vi "Compile Fully Custom Teeth.vi"(7 "Custom Device Ref":T1 format="%.0x", 8 "error in (no error)":errorcluster, 10 "Channel Descriptors in":T2, 11 "Fully custom teeth refs":T1[](array[typedef]) format="%.0x") -> (0 "error out":errorcluster, 2 "Channel Descriptors out":T2, 4 "Fully Custom Teeth":T9[](array[typedef]))   [LabVIEW 2011, in "Engine Sim System Explorer.lvlib"]
uses:
  Engine Sim System Explorer.lvlib
  <vilib>/NI Veristand/Custom Device API/Custom Device API.lvlib
  <vilib>/NI Veristand/Custom Device API/Get Item Property (U16).vi
  <vilib>/NI Veristand/Custom Device API/Get Item Property (Variant).vi
  <vilib>/NI Veristand/Custom Device API/Get Item Property (Boolean).vi
  Shared/Engine Simulation Global.vi
  Engine Simulation Shared.lvlib
  Shared/FullyCustomProfileConfig.ctl
  Shared/FullyCustomCommMode.ctl
  Shared/FullyCustomConfig.ctl
  <vilib>/NI Veristand/Custom Device API/Custom Device Item Ref.ctl
  Shared/InputChannelTypes.ctl
  <vilib>/rvi/DataTransferAndStorage/Container/Common/niFpgaDataTypeControl.ctl
  Shared/FPGA Write Descriptor.ctl
  Shared/OutputChannelTypes.ctl
  Shared/FPGA Read Descriptor.ctl
  Shared/Channel Descriptors.ctl
  Shared/Status Chan Descriptor.ctl
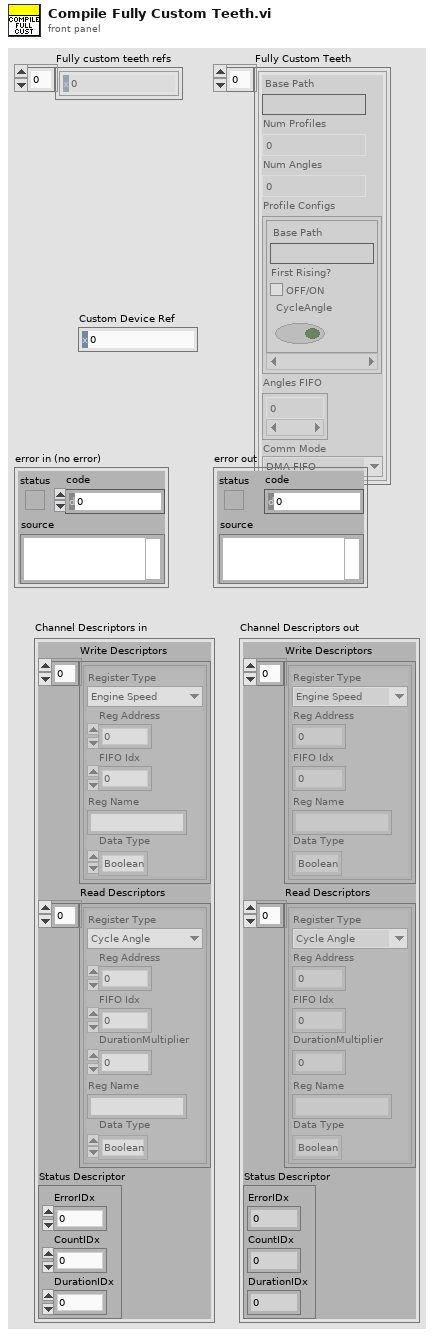
[diagram p1: front panel]
types:
  T1 = typedef "Custom Device API.lvlib/Custom Device Item Ref.ctl" = u64
  T2 = typedef "Engine Simulation Shared.lvlib/Channel Descriptors.ctl" = cluster{"Write Descriptors":T3[], "Read Descriptors":T6[], "Status Descriptor":T8}
  T3 = typedef "Engine Simulation Shared.lvlib/FPGA Write Descriptor.ctl" = cluster{"Register Type":T4, "Reg Address":u32, "FIFO Idx":i32, "Reg Name":string, "Data Type":T5}
  T4 = typedef "Engine Simulation Shared.lvlib/InputChannelTypes.ctl" = enum16{"Engine Speed", "Offset"}
  T5 = typedef "niFpgaDataTypeControl.ctl" = enum32{"Boolean", "I8", "I16", "I32", "I64", "U8", "U16", "U32", "U64", "FXP", "CustomControl"}
  T6 = typedef "Engine Simulation Shared.lvlib/FPGA Read Descriptor.ctl" = cluster{"Register Type":T7, "Reg Address":u32, "FIFO Idx":i32, "DurationMultiplier":dbl, "Reg Name":string, "Data Type":T5}
  T7 = typedef "Engine Simulation Shared.lvlib/OutputChannelTypes.ctl" = enum16{"Cycle Angle", "Crank Angle", "Time Duration", "Angle Duration", "Start Angle", "End Angle"}
  T8 = typedef "Engine Simulation Shared.lvlib/Status Chan Descriptor.ctl" = cluster{"ErrorIDx":i32, "CountIDx":i32, "DurationIDx":i32}
  T9 = typedef "Engine Simulation Shared.lvlib/FullyCustomConfig.ctl" = cluster{"Base Path":string, "Num Profiles":u8, "Num Angles":u8, "Profile Configs":T10[], "Angles FIFO":u64[], "Comm Mode":T11}
  T10 = typedef "Engine Simulation Shared.lvlib/FullyCustomProfileConfig.ctl" = cluster{"Base Path":string, "First Rising?":bool, "CycleAngle":bool}
  T11 = typedef "Engine Simulation Shared.lvlib/FullyCustomCommMode.ctl" = enum16{"DMA FIFO", "FP Data Transfer"}
  T12 = typedef "Custom Device API.lvlib/Custom Device Item Info.ctl" = cluster{"Name":string, "Is Channel":bool, "GUID":string}
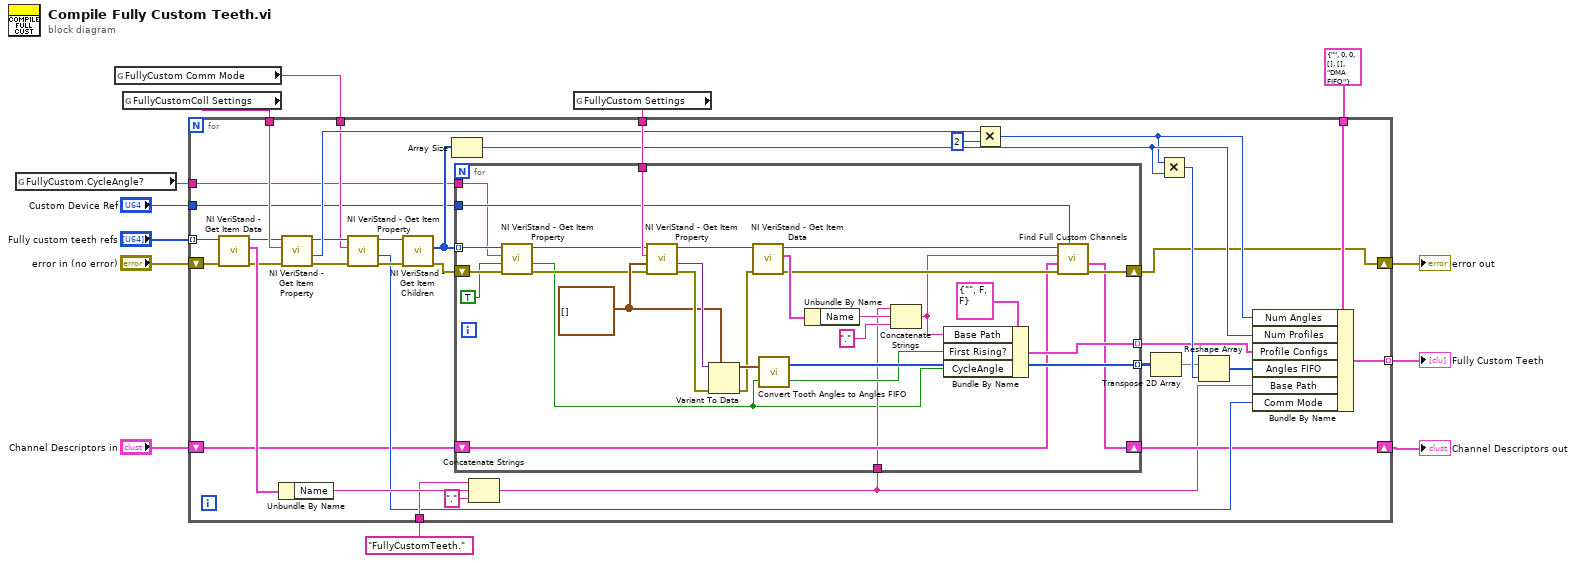
[diagram p0: block diagram]
diagram:
  n1 = global read "Engine Simulation Global.vi" "FullyCustom.CycleAngle?"() -> (w13:string)
  n2 = global read "Engine Simulation Global.vi" "FullyCustom Comm Mode"() -> (w12:string)
  n3 = global read "Engine Simulation Global.vi" "FullyCustomColl Settings"() -> (w6:string)
  n4 = global read "Engine Simulation Global.vi" "FullyCustom Settings"() -> (w7:string)
  n5 = for {
    shift-right: [w19] -> w10
    shift-left: "error in (no error)" -> [w41]
    tunnel: "Fully custom teeth refs" -> [w40] mode=indexing
    tunnel: w6 -> [w48]
    tunnel: w7 -> [w46]
    tunnel: T9 {"Base Path"="", "Num Profiles"=0, "Num Angles"=0, "Profile Configs"=[], "Angles FIFO"=[], "Comm Mode"=enum."DMA FIFO"} ("FullyCustom Config") -> [w38]
    tunnel: "FullyCustomTeeth." ("string") -> [w31]
    tunnel: [w20] -> w11 mode=indexing
    tunnel: w12 -> [w24]
    tunnel: w13 -> [w14]
    shift-right: [w17] -> w2
    shift-left: "Channel Descriptors in" -> [w18]
    tunnel: "Custom Device Ref" -> [w15]
    n6 = call <vilib>:"NI VeriStand - Get Item Data.vi"("error in (no error)"=w41, "Item Ref in"=w40) -> ("error out"=w22:errorcluster, "Item Info"=w39:T12, "Item Ref out"=w21:T1)  [unwired: 6 in, 1 out]
    n7 = Unbundle By Name(w39) -> ("Name"=w33:string)
    n8 = call-poly <vilib>:"NI VeriStand - Get Item Property.vi"("error in (no error)"=w22, "Property Name"=w48, "Item Ref in"=w21) -> ("error out"=w28:errorcluster, "Value"=w36:u16, "Item Ref out"=w25:T1)  [unwired: 5 in, 1 out]
    n9 = call-poly <vilib>:"NI VeriStand - Get Item Property.vi"("error in (no error)"=w28, "Property Name"=w24, "Item Ref in"=w25) -> ("error out"=w27:errorcluster, "Value"=w23:u16, "Item Ref out"=w26:T1)  [unwired: 5 in, 1 out]
    n10 = call <vilib>:"NI VeriStand - Get Item Children.vi"("error in (no error)"=w27, "Item Ref in"=w26) -> ("error out"=w47:errorcluster, "Child Refs"=w45:T1[])  [unwired: 6 in, 2 out]
    n11 = Array Size(array=w45) -> (size(s)=w35:i32)
    n12 = Concatenate Strings(w31, w33, "." ("string")) -> (w16:string)
    n13 = for {
      tunnel: w45 -> [w53] mode=indexing
      tunnel: w46 -> [w76]
      tunnel: [w69] -> w44 mode=indexing
      shift-right: [w60] -> w19
      shift-left: w47 -> [w77]
      tunnel: [w66] -> w34 mode=indexing
      shift-right: [w58] -> w17
      shift-left: w18 -> [w59]
      tunnel: w16 -> [w57]
      tunnel: w15 -> [w55]
      tunnel: w14 -> [w51]
      w64 = cluster{"Falling Edge":dbl, "Rising Edge":dbl}[] [] ("Tooth Angles")
      n14 = call-poly <vilib>:"NI VeriStand - Get Item Property.vi"("error in (no error)"=w77, "Default Value"=TRUE, "Property Name"=w51, "Item Ref in"=w53) -> ("error out"=w54:errorcluster, "Value"=w49:bool, "Item Ref out"=w52:T1)  [unwired: 4 in, 1 out]
      n15 = call-poly <vilib>:"NI VeriStand - Get Item Property.vi"("error in (no error)"=w54, "Default Value"=w64, "Property Name"=w76, "Item Ref in"=w52) -> ("error out"=w73:errorcluster, "Value"=w75:variant, "Item Ref out"=w72:T1)  [unwired: 4 in, 1 out]
      n16 = Variant To Data(error in=w73, type=w64, Variant=w75) -> (data=w74:cluster{"Falling Edge":dbl, "Rising Edge":dbl}[], error out=w70:errorcluster)
      n17 = call <vilib>:"NI VeriStand - Get Item Data.vi"("error in (no error)"=w70, "Item Ref in"=w72) -> ("error out"=w63:errorcluster, "Item Info"=w71:T12, "Item Ref out"=w61:T1)  [unwired: 6 in, 1 out]
      n18 = call "Convert Tooth Angles to Angles FIFO.vi"("Cycle Angle?"=w49, "Tooth Angles"=w74) -> ("First Rising?"=w65:bool, "FullyCustomProfile"=w69:u64[])
      n19 = Unbundle By Name(w71) -> ("Name"=w68:string)
      n20 = Concatenate Strings(w57, w68, "." ("string")) -> (w56:string)
      n21 = Bundle By Name(cluster=T10 {"Base Path"="", "First Rising?"=FALSE, "CycleAngle"=FALSE} ("Profile Config"), "Base Path"=w56, "First Rising?"=w65, "CycleAngle"=w49) -> (w66:T10)
      n22 = call "Find Full Custom Channels.vi"("Custom Device Ref"=w55, "error in (no error)"=w63, "Channel Descriptors in"=w59, "Base path"=w56, "Full Custom ref"=w61) -> ("error out"=w60:errorcluster, "Channel Descriptors out"=w58:T2)  [unwired: 5 in]
    }
    n23 = Multiply(x=w36, y=u16 2) -> (x*y=w30:u16)
    n24 = Transpose 2D Array(2D array=w44) -> (transposed array=w42:u64[][])
    n25 = Multiply(x=w30, y=w35) -> (x*y=w43:i32)
    n26 = Reshape Array(w42, w43) -> (w37:u64[])
    n27 = Bundle By Name(cluster=w38, "Num Angles"=w30, "Num Profiles"=w35, "Profile Configs"=w34, "Angles FIFO"=w37, "Base Path"=w16, "Comm Mode"=w23) -> (w20:T9)
  }
  "Fully Custom Teeth" <- w11
  "error out" <- w10
  "Channel Descriptors out" <- w2
